vi "Call Subpanel VI.vi"(8 "error in (no error)":errorcluster, 10 "VI Refnum":refnum<vi>, 11 "Configuration in":refnum<class "Configuration.lvclass">) -> (0 "error out":errorcluster, 3 "Configuration out":refnum<class "Configuration.lvclass">)   [LabVIEW 2016, in "Configuration.lvlib" / "Configuration.lvclass"]
uses:
  <userlib>/Configuration Dialog Actor/Configuration.lvclass
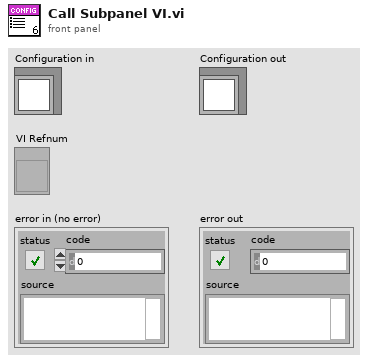
[diagram p1: front panel]
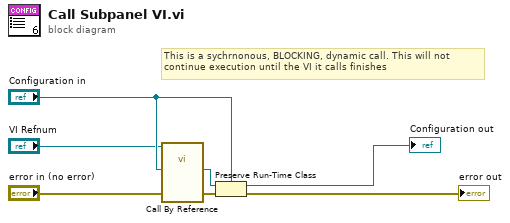
[diagram p0: block diagram]
diagram:
  # "This is a sychrnonous, BLOCKING, dynamic call. This will not\ncontinue execution until the VI it calls finishes"
  n1 = call-by-ref "?"(reference="VI Refnum", "error in (no error)"="error in (no error)", "Configuration in"="Configuration in") -> ("error out"=w6:errorcluster, "Configuration out"=w4:refnum<class "Configuration.lvclass">)  [unwired: 9 in, 2 out]
  n2 = Preserve Run-Time Class(object in=w4, error in=w6, 2:"Configuration in") -> (object out=→"Configuration out":refnum<class "Configuration.lvclass">, error out=→"error out":errorcluster)
